vi "CalibracaoDosSensores.vi"(5 "Pump and sensor data in":dbl[](array[numeric])) -> (2 "Pump and sensor data out":dbl[](array[numeric]))   [LabVIEW 2015]
doc: "This VI calibrates sensors values."
panel:
  in  "y 2":dbl[](array[numeric])=[0.0, 0.0, 0.0, 0.0]
  in  "y":dbl[](array[numeric])=[2.5, 2.5, 2.5, 2.5]
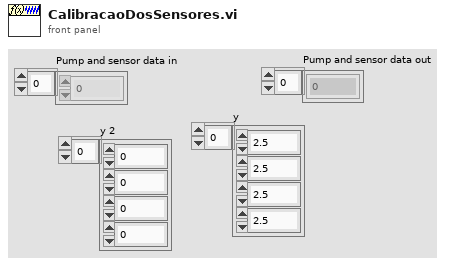
[diagram p1: front panel]
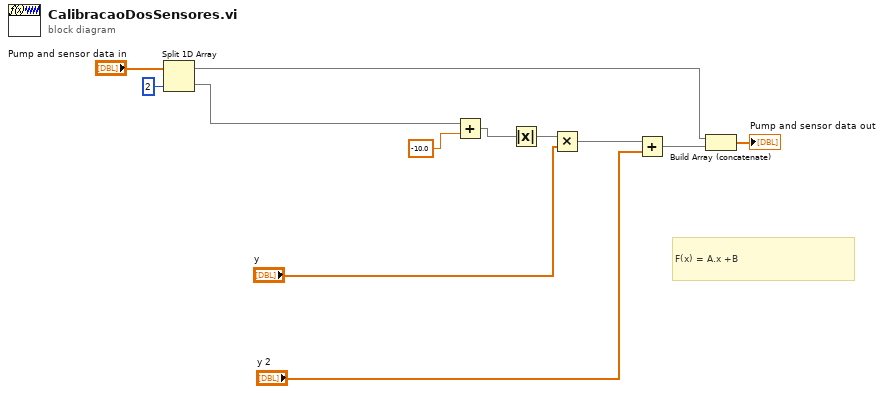
[diagram p0: block diagram]
diagram:
  # "F(x) = A.x +B"
  n1 = Split 1D Array(array="Pump and sensor data in", index=2) -> (first subarray=w3:dbl[], second subarray=w6:dbl[])
  n2 = Add(x=w6, y=-10.0) -> (x+y=w9:dbl[])
  n3 = Absolute Value(x=w9) -> (abs(x)=w4:dbl[])
  n4 = Multiply(x=w4, y="y") -> (x*y=w12:dbl[])
  n5 = Add(x=w12, y="y 2") -> (x+y=w2:dbl[])
  n6 = Build Array (concatenate)(w3, w2) -> (→"Pump and sensor data out":dbl[])
